vi "AR Drone Controller with PS3 Support.vi"() -> ()   [LabVIEW 2014]
doc: "Very simple example showing how to use the base VIs to control the AR Drone and receive and display navigation data."
uses:
  Control 1.ctl
  <vilib>/LVH/AR Drone Toolkit/Decode NavData/Typedefs/NavData Demo.ctl
  <vilib>/picture/picture.llb/Draw True-Color Pixmap.vi
  <vilib>/LVH/AR Drone Toolkit/AR Drone.lvlib
  Drone Project/AR Drone Toolkit (BETA)/Decode Video/2.0/Decode20Video.dll
panel:
  out "error out":errorcluster
  in  "Reset":bool
  out "vid":errorcluster
  out "nav":errorcluster
  out "ctr":errorcluster
  out "vid":i32
  out "nav":i32
  out "ctr":i32
  out "Video Data Out (2.0)":u8[](array[numeric])
  in  "Emergency Landing":bool
  in  "Takeoff/Land":bool
  out "Video Stream":picture
  in  "Tab Control":enum32{"Setup", "Control", "Navigation"}(tab)
  out "input device":T1
  in  "controller ID":i32
  in  "GO!":bool
  in  "Ignore errors":bool
  in  "Setup Parameters":T2={"Drone IP address"="192.168.1.1", "Home IP address"="192.168.1.2", "Flight Mode"=enum."INDOOR MODE", "Mounted Hull"=enum."INDOOR HULL", "Video Camera"=2, "Max Altitude (m)"=3.0, "Max Pitch and Roll Angle (deg)"=10.0, "Max Vertical Speed (m/s)"=0.7, "Max Yaw Speed (deg/s)"=100.0} {"Video Camera" items=["Bottom Camera"=1, "Front Camera"=0, "Front in Bottom"=3, "Bottom in Front"=2]}
  out "Control cluster":T3 {"Roll" scale=-1.0..1.0; "Pitch" scale=-1.0..1.0; "Vertical Speed" scale=-1.0..1.0; "Yaw Speed" scale=-1.0..1.0}
  out "Battery Remaining":T4 scale=0.0..100.0
  out "Waveform Chart":u32(graph)
  out "XY Graph":cluster{"Y":dbl[], "Y":dbl[]}[](graph)
  out "NavData Out":T5
  in  "milliseconds to wait":u32=50
  in  "STOP":bool
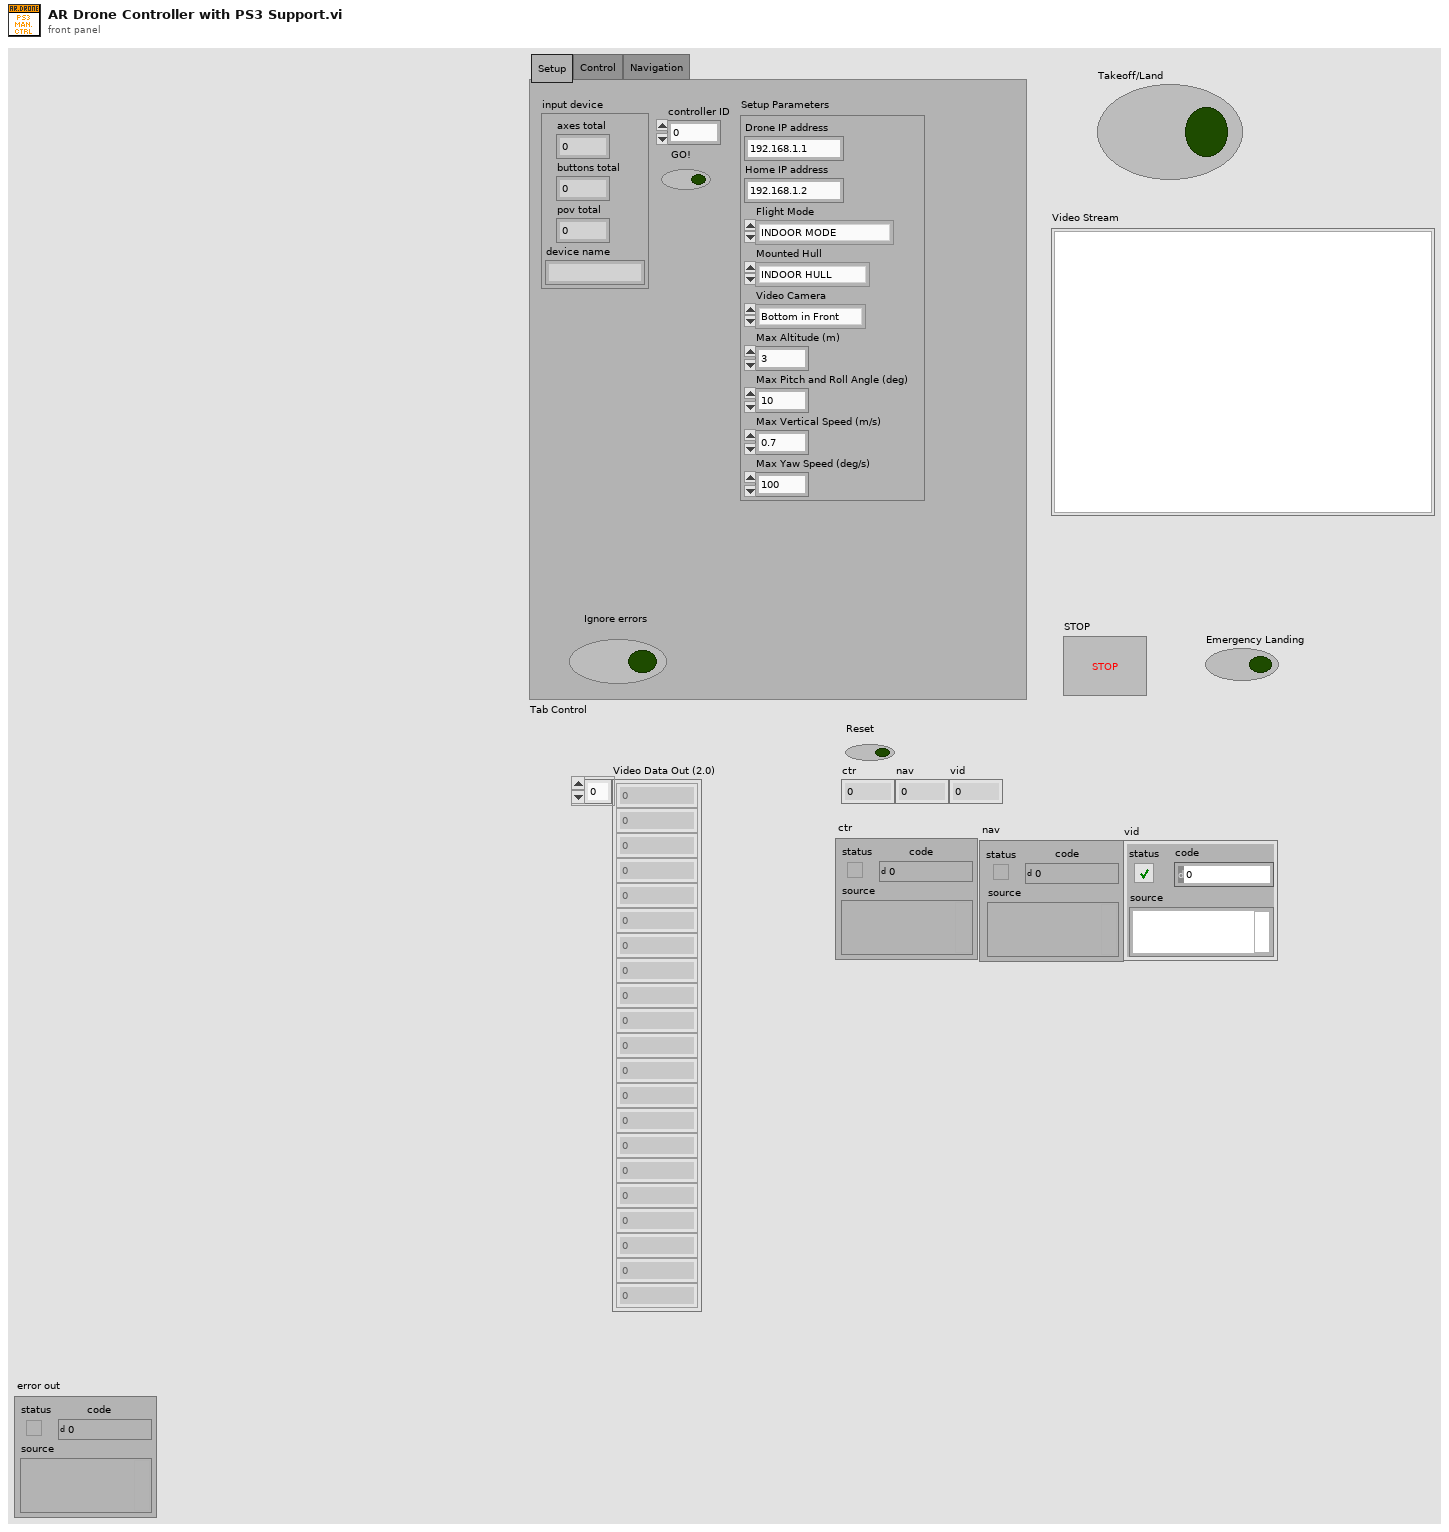
[diagram p1: front panel]
types:
  T1 = cluster{"axes total":u32, "buttons total":u32, "pov total":u32, "device name":string}
  T2 = cluster{"Drone IP address":string, "Home IP address":string, "Flight Mode":enum8{"OUTDOOR MODE", "INDOOR MODE"}, "Mounted Hull":enum8{"OUTDOOR HULL", "INDOOR HULL"}, "Video Camera":u8, "Max Altitude (m)":sgl, "Max Pitch and Roll Angle (deg)":sgl, "Max Vertical Speed (m/s)":sgl, "Max Yaw Speed (deg/s)":sgl}
  T3 = cluster{"Roll":dbl, "Pitch":dbl, "Vertical Speed":dbl, "Yaw Speed":dbl}
  T4 = typedef "Control 1.ctl" = dbl
  T5 = typedef "AR Drone.lvlib/NavData Demo.ctl" = cluster{"control state":enum32{"DEFAULT", "INIT", "LANDING", "FLYING", "HOVERING", "TEST", "TRANS_TAKEOFF", "TRANS_GOTOFIX", "TRANS_LANDING"}, "battery percentage":u32, "pitch (deg)":sgl, "roll (deg)":sgl, "yaw (deg)":sgl, "altitude (cm)":u32, "vx (cm/s)?":sgl, "vy (cm/s)?":sgl, "vz (cm/s)?":sgl, "detection cam type":u32}
  T6 = typedef "AR Drone.lvlib/AR Drone Resource.ctl" = cluster{"UDP Control Connection":refnum<k16>, "UDP NavData Connection":refnum<k16>, "UDP Video Connection (Drone 1.0)":refnum<k16>, "TCP Video Connection (Drone 2.0)":refnum<k5>, "TCP Control Port Connection":refnum<k5>, "Drone IP address":string, "Drone Command Port":u16, "Drone NavData Port":u16, "Drone Vid Stream Port":u16, "Drone TCP Control Port":u16, "Home IP address":string, "Home Command Port":u16, "Home NavData Port":u16, "Home Vid Stream Port":u16, "Drone Version":i32}
  T7 = cluster{"Hover":bool, bool, "Emergency Landing":bool, "button 4":bool, "button 5":bool, "button 6":bool, "button 7":bool, "button 8":bool}
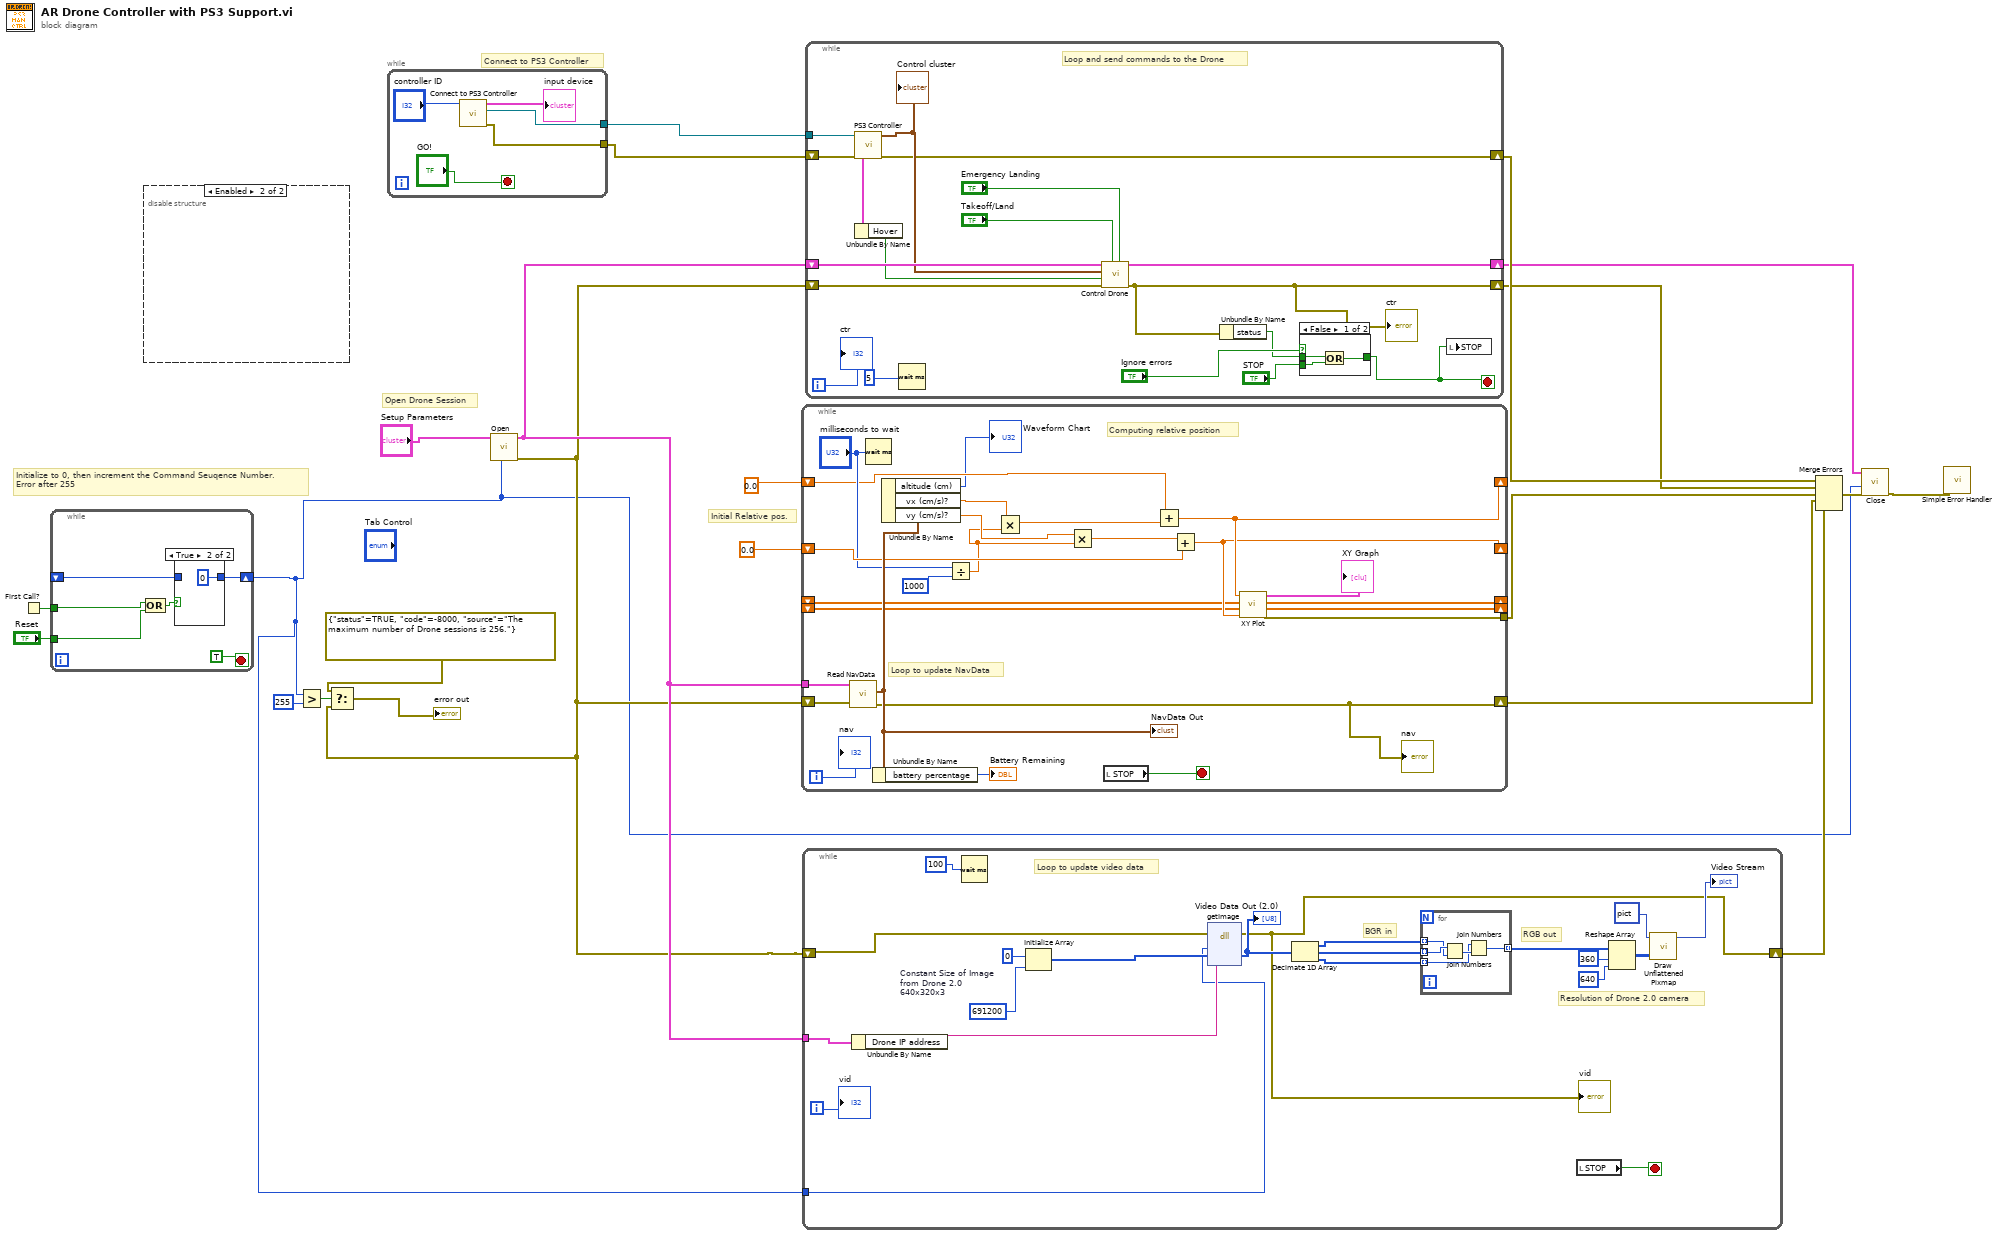
[diagram p0: block diagram]
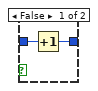
[diagram p2: hidden frame]
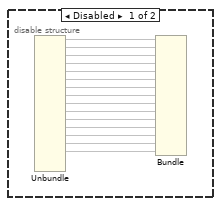
[diagram p3: hidden frame]
diagram:
  # "Initialize to 0, then increment the Command Seuqence Number.\nError after 255"
  # "Initial Relative pos."
  # "Connect to PS3 Controller"
  # "Open Drone Session"
  n1 = First Call?() -> (First Call?: T/F=w8:bool)
  n2 = while {
    tunnel: w8 -> [w24]
    shift-right: [w27] -> w1
    shift-left: _ -> [w26]
    tunnel: "Reset" -> [w23]
    stop <- TRUE stop-if-true
    n3 = Compound Arithmetic op=OR(w24, w23) -> (w25:bool)
    n4 = case shown="True" w25 {
      tunnel: [w29 0] -> w27
      tunnel: w26 -> [w30 _]
      frame False {
        n5 = Increment(x=w30) -> (x+1=w29:i32)
      }
      frame True {
      }
    }
  }
  n6 = disable-structure shown="Enabled" {
    frame Disabled {
      n7 = Unbundle() -> ("UDP Control Connection"=w46, "UDP NavData Connection"=w45, "UDP Video Connection (Drone 1.0)"=w44, "TCP Video Connection (Drone 2.0)"=w43, "TCP Control Port Connection"=w42, "Drone IP address"=w41, "Drone Command Port"=w40, "Drone NavData Port"=w39, "Drone Vid Stream Port"=w38, "Drone TCP Control Port"=w37, "Home IP address"=w36, "Home Command Port"=w35, "Home NavData Port"=w34, "Home Vid Stream Port"=w33, "Drone Version"=w32)  [unwired: 1 in, 2 out]
      n8 = Bundle(w46, w45, w44, w43, w42, w41, w40, w39, w38, w37, w36, w35, w34, w33, w32) -> ()  [unwired: 1 in, 1 out]
    }
    frame Enabled {
    }
  }
  n9 = Greater?(x=w1, y=255) -> (0:w5:bool)
  n10 = while {
    tunnel: [w51] -> w19
    tunnel: [w47] -> w18
    stop <- "GO!" stop-if-true
    n11 = call "Connect to PS3 Controller.vi"("device ID"="controller ID") -> ("error out"=w47:errorcluster, "device ID 2"=w51:refnum<k1>, "element"=→"input device":T1)  [unwired: 7 in]
  }
  n12 = call <vilib>:"Open.vi"("drone index"=w1, "Setup Parameters"="Setup Parameters") -> ("error out"=w2:errorcluster, "AR Drone Resource"=w9:T6)  [unwired: 8 in]
  n13 = Select(t=errorcluster {"status"=TRUE, "code"=-8000, "source"="The maximum number of Drone sessions is 256."}, s=w5, f=w2) -> (s? t:f=→"error out":errorcluster)
  n14 = while {
    shift-right: [w52] -> w13
    shift-left: w2 -> [w61]
    shift-right: [w72] -> _
    shift-left: 0.0 -> [w60]
    shift-right: [w71] -> _
    shift-left: 0.0 -> [w74]
    tunnel: [w62] -> w14
    shift-right: [w68] -> _
    shift-left: _ -> [w70]
    shift-right: [w67] -> _
    shift-left: _ -> [w69]
    tunnel: w9 -> [w54]
    i -> [w53]
    stop <- w66 stop-if-true
    # "Computing relative position"
    # "Loop to update NavData"
    n15 = call <vilib>:"Read NavData.vi"("error in (no error)"=w61, "AR Drone Resource"=w54) -> ("error out"=w52:errorcluster, "NavData Out"=w75:T5)  [unwired: 7 in, 1 out]
    "NavData Out" <- w75
    "nav" <- w52
    n16 = Wait (ms)(milliseconds to wait="milliseconds to wait") -> ()  [unwired: 1 out]
    n17 = Unbundle By Name(w75) -> ("battery percentage"=→"Battery Remaining":u32)
    n18 = Unbundle By Name(w75) -> ("altitude (cm)"=→"Waveform Chart":u32, "vx (cm/s)?"=w57:sgl, "vy (cm/s)?"=w56:sgl)
    n19 = Divide(x="milliseconds to wait", y=u32 1000) -> (x/y=w55:dbl)
    n20 = Multiply(x=w57, y=w55) -> (x*y=w63:dbl)
    n21 = Multiply(x=w56, y=w55) -> (x*y=w58:dbl)
    n22 = local read "STOP"() -> (w66:bool)
    n23 = Add(x=w60, y=w63) -> (x+y=w72:dbl)
    n24 = Add(x=w58, y=w74) -> (x+y=w71:dbl)
    n25 = call "XY Plot.vi"("X"=w72, "X array"=w70, "Y array"=w69, "Y"=w71) -> ("XY Graph"=→"XY Graph":cluster{"Y":dbl[], "Y":dbl[]}[], "X array"=w68:dbl[], "Y array"=w67:dbl[], "error out"=w62:errorcluster)  [unwired: 2 in]
    "nav" <- w53
  }
  n26 = while {
    tunnel: w9 -> [w81]
    tunnel: w1 -> [w77]
    shift-right: [w78] -> w10
    shift-left: w2 -> [w92]
    i -> [w79]
    stop <- w97 stop-if-true
    w95 = 691200  # Constant Size of Image from Drone 2.0 640x320x3
    # "Resolution of Drone 2.0 camera"
    # "RGB out"
    # "BGR in"
    # "Loop to update video data"
    n27 = Unbundle By Name(w81) -> ("Drone IP address"=w80:string)
    n28 = Wait (ms)(milliseconds to wait=u32 100) -> ()  [unwired: 1 out]
    n29 = Initialize Array(u8 0 ("dimension size"), w95) -> (w93:u8[])
    n30 = dll-call lib="E:/Dropbox/UTCN/Summer 2015/Drone Project/AR Drone Toolkit (BETA)/Decode Video/2.0/Decode20Video.dll" fn="getImage"(error in=w92, "Index"=w77, "ImgData"=w93, "IP Address"=w80) -> (error out=w78:errorcluster, "ImgData"=w83:u8[])  [unwired: 5 in, 1 out]
    "Video Data Out (2.0)" <- w83
    "vid" <- w78
    n31 = Decimate 1D Array(w83) -> (w86:u8[], w85:u8[], w84:u8[])
    n32 = for {
      tunnel: [w101] -> w91 mode=indexing
      tunnel: w86 -> [w99] mode=indexing
      tunnel: w85 -> [w100] mode=indexing
      tunnel: w84 -> [w98] mode=indexing
      n33 = Join Numbers(hi=w100, lo=w99) -> ((hi.lo)=w102:u16)
      n34 = Join Numbers(hi=w98, lo=w102) -> ((hi.lo)=w101:u32)
    }
    n35 = local read "STOP"() -> (w97:bool)
    n36 = Reshape Array(w91, 360 ("dimension size"), 640 ("dimension size")) -> (w90:u32[][])
    n37 = call-poly <vilib>:"Draw Unflattened Pixmap.vi"("picture"=picture data[5B], "data (RGB format)"=w90) -> ("new picture"=→"Video Stream":picture)  [unwired: 7 in]
    "vid" <- w79
  }
  n38 = while {
    shift-right: [w119] -> w12
    shift-left: w9 -> [w120]
    tunnel: w19 -> [w113]
    shift-right: [w103] -> w15
    shift-left: w2 -> [w118]
    shift-right: [w116] -> w16
    shift-left: w18 -> [w112]
    i -> [w104]
    stop <- w108 stop-if-true
    # "Loop and send commands to the Drone"
    n39 = call "PS3 Controller.vi"("error in (no error)"=w112, "device ID"=w113) -> ("error out"=w116:errorcluster, "Buttons"=w115:T7, "Control cluster"=w117:T3)  [unwired: 6 in, 1 out]
    "Control cluster" <- w117
    n40 = Unbundle By Name(w115) -> ("Hover"=w111:bool)
    n41 = Wait (ms)(milliseconds to wait=u32 5) -> ()  [unwired: 1 out]
    n42 = call <vilib>:"Control Drone.vi"("Emergency Landing"="Emergency Landing", "Takeoff/Land"="Takeoff/Land", "error in (no error)"=w118, "Hover"=w111, "Control Cluster"=w117, "AR Drone Resource"=w120) -> ("error out"=w103:errorcluster, "AR Drone Resource Out"=w119:T6)  [unwired: 4 in]
    "ctr" <- w103
    n43 = Unbundle By Name(w103) -> ("status"=w107:bool)
    n44 = case shown="False" "Ignore errors" {
      tunnel: w107 -> [w122 _]
      tunnel: [w123 w124] -> w108
      tunnel: "STOP" -> [w121 w124]
      frame False {
        n45 = Or(x=w122, y=w121) -> (x .or. y?=w123:bool)
      }
      frame True {
      }
    }
    n46 = local write "STOP"(w108) -> ()
    "ctr" <- w104
  }
  n47 = Merge Errors(w16, w15, w14, w13, w10) -> (w17:errorcluster)
  n48 = call <vilib>:"Close.vi"("error in (no error)"=w17, "Index"=w1, "AR Drone Resource"=w12) -> ("error out"=w22:errorcluster)  [unwired: 8 in]
  n49 = call <vilib>:"Simple Error Handler.vi"("error in (no error)"=w22) -> ()  [unwired: 4 in, 5 out]
